vi "Read Lossy.vi"(0 "Wait for Next? (F)":bool, 2 "FlexChannel":T2, 3 "Wait Timeout mS (-1)":i32=-1) -> (1 "Updated":timestamp, 4 "Sequence":u32, 5 "Timed Out?":bool, 7 "Value":T1, 8 "Closed?":bool)   [LabVIEW 2020, in "Flex.lvlib"]
doc: "Allows reading tag-like data from the channel. This reader endpoint will behave closer to a notifier if the <b>Wait for Next</b> input is set to true otherwise it will return the latest value that has been set. The Timeout will only apply when Wait for Next is set. The <b>Closed</b> output will return true when the writer has been closed and can be used to close down the reader's loop."
uses:
  Flex.lvlib
  ))Channel.ctl
  Element.ctl
  ChannelOp.ctl
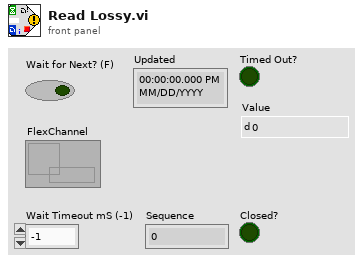
[diagram p1: front panel]
types:
  T1 = typedef "Flex.lvlib/Element.ctl" = dbl
  T2 = typedef "Flex.lvlib/))Channel.ctl" = refnum<queue>
  T3 = typedef "Flex.lvlib/ChannelOp.ctl" = enum16{"Get Refs", "Init", "Close", "Probe", "New Queue", "Remove Queue"}
  T4 = typedef "Flex.lvlib/Channel Data.ctl" = cluster{"Element":refnum<data-value>, "Queue Refs":refnum<data-value>, "Update":refnum<k4>}
  T5 = typedef "Flex.lvlib/Element Info.ctl" = cluster{"Value":T1, "Updated":timestamp, "Sequence":u32}
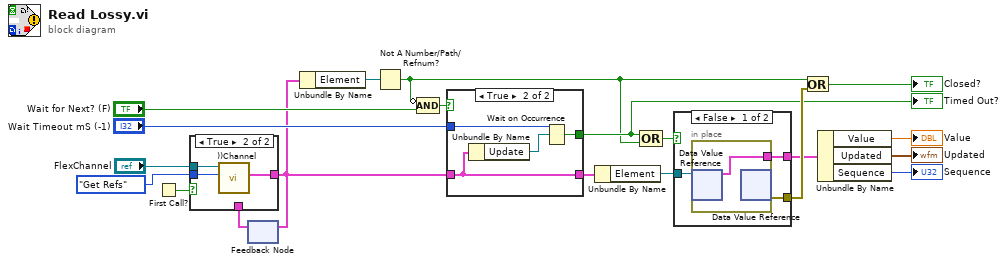
[diagram p0: block diagram]
diagram:
  n1 = First Call?() -> (First Call?: T/F=w17:bool)
  n2 = feedback #1() -> (w16:T4)  [unwired: 1 in]
  n3 = case shown="True" w17 {
    tunnel: "FlexChannel" -> [_ w24]
    tunnel: ChannelOp."Get Refs" ("channelOp") -> [_ w23]
    tunnel: [w21 w22] -> w10
    tunnel: w16 -> [w21 _]
    frame False {
    }
    frame True {
      n4 = call "))Channel.vi"("channelOp"=w23, "channel in"=w24) -> ("Channel Data"=w22:T4)  [unwired: 6 in, 3 out]
    }
  }
  n5 = feedback-in #1(w10) -> ()
  n6 = Unbundle By Name(w10) -> ("Element"=w12:refnum<data-value>)
  n7 = Not A Number/Path/Refnum?(number/path/refnum=w12) -> (NaN/Path/Refnum?=w8:bool)
  n8 = Compound Arithmetic op=AND(invert w8, "Wait for Next? (F)") -> (w9:bool)
  n9 = case shown="True" w9 {
    tunnel: w10 -> [w25 w26]
    tunnel: "Wait Timeout mS (-1)" -> [_ w28]
    tunnel: [_ w27] -> w13
    tunnel: [w25 w26] -> w7
    frame False {
    }
    frame True {
      n10 = Unbundle By Name(w26) -> ("Update"=w29:refnum<k4>)
      n11 = Wait on Occurrence(2:w29, 3:w28) -> (0:w27:bool)  [unwired: 1 in]
    }
  }
  "Timed Out?" <- w13
  n12 = Unbundle By Name(w7) -> ("Element"=w6:refnum<data-value>)
  n13 = Compound Arithmetic op=OR(w13, w8) -> (w11:bool)
  n14 = case shown="False" w11 {
    tunnel: [w32 _] -> w4
    tunnel: w6 -> [w31 _]
    tunnel: [w30 _] -> w20
    frame False {
      n15 = in-place {
        in-place-border: [w33] -> w32
        n16 = in-place-dvr #2(w31) -> (w33:T5)  [unwired: 1 out]
        n17 = in-place-dvr #2() -> (w30:errorcluster)  [unwired: 1 in, 1 out]
      }
    }
    frame True {
    }
  }
  n18 = Or(x=w8, y=w20) -> (x .or. y?=→"Closed?":bool)
  n19 = Unbundle By Name(w4) -> ("Value"=→"Value":T1, "Updated"=→"Updated":timestamp, "Sequence"=→"Sequence":u32)
